vi "Query Generator ARB File Version.vi"(8 "error in (no error)":errorcluster, 10 "Instance (1)":i32=1 format="%.0g", 11 "VISA resource name":refnum<visa-resource-name>) -> (0 "error out":errorcluster, 2 "File Version":string, 3 "VISA resource name out":refnum<visa-resource-name>)   [LabVIEW 2020, in "Rohde&Schwarz CMXP GPRF.lvlib"]
doc: "Queries the version of the loaded waveform file.\n\nAttribute:\nRSCMXPGPRF_ATTR_ARB_FILE_VERSION\n\nRemote-control command:\nSOURce:GPRF:GEN<i>:ARB:FILE:VERSion?"
uses:
  <instrlib>/Rohde&Schwarz CMXP GPRF/Rohde&Schwarz CMXP GPRF.lvlib
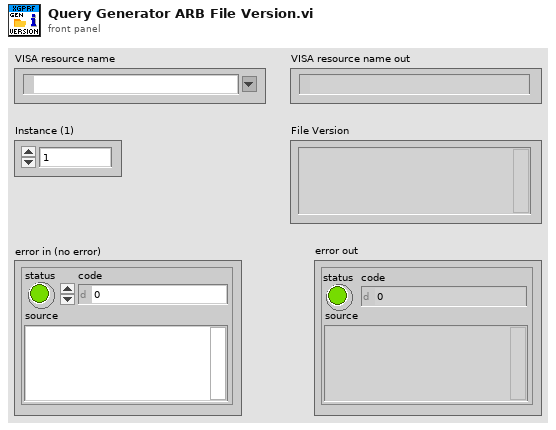
[diagram p1: front panel]
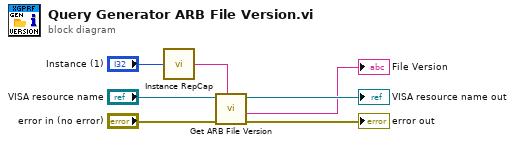
[diagram p0: block diagram]
diagram:
  n1 = call <instrlib>:"Instance RepCap.vi"("Instance in"="Instance (1)") -> ("Instance out"=w7:string)
  n2 = call "Get ARB File Version"("Repeated Capabilities"=w7, "error in (no error)"="error in (no error)", "instrument handle"="VISA resource name") -> ("error out"=→"error out":errorcluster, "ARB File Version"=→"File Version":string, "instrument handle out"=→"VISA resource name out":refnum<visa-resource-name>)  [unwired: 6 in]
